vi "Wait for Magnet Setpoint.vi"(6 "Axis":T1=enum."Z", 8 "error in (no error)":errorcluster, 9 "Tolerance (T)":dbl, 10 "Setpoint (T)":dbl, 11 "Instrument.Cryostat in":refnum<class "Instrument.Cryostat.lvclass">) -> (0 "error out":errorcluster, 3 "Instrument.Cryostat out":refnum<class "Instrument.Cryostat.lvclass">)   [LabVIEW 2019, in "Instrument.Cryostat.lvclass"]
uses:
  Instrument.Cryostat.lvclass
  Typedefs/Magnet Axis--Enum.ctl
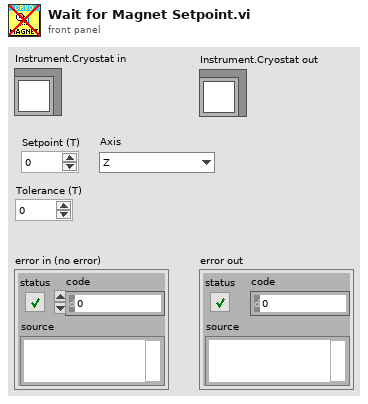
[diagram p1: front panel]
types:
  T1 = typedef "Instrument.Cryostat.lvclass/Magnet Axis--Enum.ctl" = enum16{"X", "Y", "Z"}
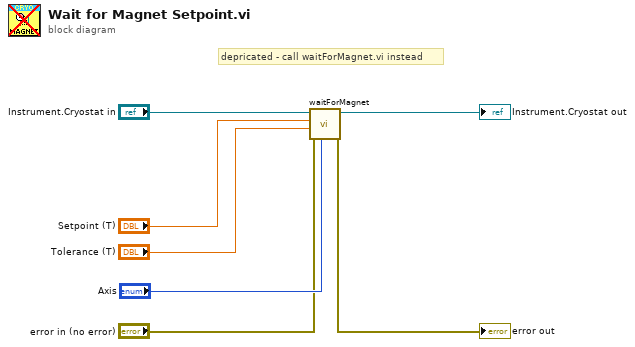
[diagram p0: block diagram]
diagram:
  # "depricated - call waitForMagnet.vi instead"
  n1 = call "waitForMagnet.vi"("Axis"="Axis", "error in (no error)"="error in (no error)", "Tolerance (T)"="Tolerance (T)", "Setpoint (T)"="Setpoint (T)", "Instrument.Cryostat in"="Instrument.Cryostat in") -> ("error out"=→"error out":errorcluster, "Instrument.Cryostat out"=→"Instrument.Cryostat out":refnum<class "Instrument.Cryostat.lvclass">)  [unwired: 5 in]
